vi "Scope Settings Dialog.vi"(11 "Scope Parameters":T1[](array[typedef]) {"Max input frequency" format="%#_6p Hz"; "Input impedance" items=["1 mega ohm"=0, "50 ohms"=2]; "Vertical coupling" items=["AC", "DC", "Ground"]; "Reference position" format="%#_6g %%"; "Min sample rate" format=" %#_6p S/s"}) -> (3 "Scope Parameters out":T1[](array[typedef]) {"Input impedance" items=["1 mega ohm"=0, "50 ohms"=2]; "Vertical coupling" items=["AC", "DC", "Ground"]; "Reference position" format="%#_6g %%"; "Min sample rate" format=" %#_6p S/s"})   [LabVIEW 2021, in "PMIC Common.lvlib"]
uses:
  PMIC Common.lvlib
  controls/UI Scope Parameters.ctl
panel:
  # "Horizontal"
  # "Vertical"
  # "Horizontal"
  # "Vertical"
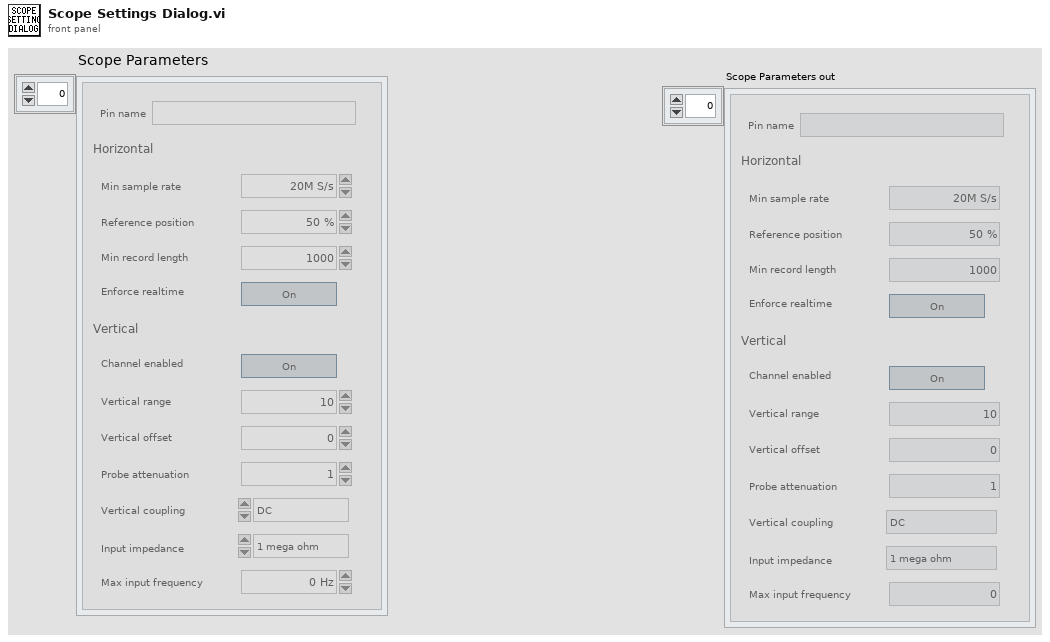
[diagram p1: front panel]
types:
  T1 = typedef "PMIC Common.lvlib/UI Scope Parameters.ctl" = cluster{"Pin name":string, "Vertical range":dbl, "Vertical offset":dbl, "Probe attenuation":dbl, "Vertical coupling":i32, "Channel enabled":bool, "Input impedance":u32, "Max input frequency":dbl, "Min sample rate":dbl, "Reference position":dbl, "Min record length":i32, "Enforce realtime":bool}
  T2 = enum32{"Invalid", "Standard", "Closed", "Hidden", "Minimized", "Maximized"}
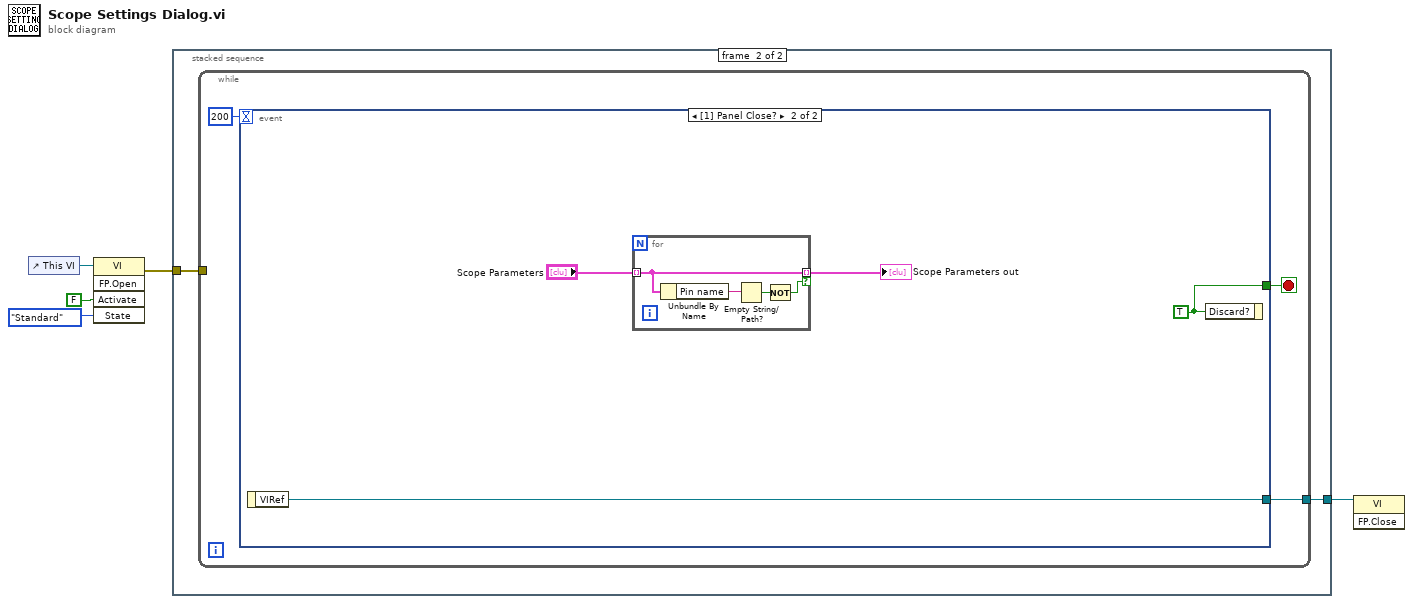
[diagram p0: block diagram]
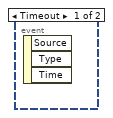
[diagram p3: hidden frame]
diagram:
  n1 = control-ref of="This VI"() -> (w5:refnum<vi>)
  n2 = invoke class="VI" method="FP.Open"(reference=w5, "Activate"=FALSE ("Activate?"), "State"=T2."Standard") -> (error out=w2:errorcluster)  [unwired: 2 in, 4 out]
  n3 = stacked-sequence {
    tunnel: w2 -> [_ w7]
    tunnel: [_ w6] -> w1
    frame #0 {
    }
    frame #1 {
      n4 = while {
        tunnel: [w8] -> w6
        tunnel: w7 -> [_]
        stop <- w10 stop-if-true
        n5 = event shown="[1] Panel Close?" {
          selector: _ -> [_ _]
          dyn-events: _ -> [_ _]
          timeout: 200 -> [_ _]
          tunnel: [_ w13] -> w10
          tunnel: [_ w14] -> w8
          event Timeout {
            n6 = event-data() -> ()  [unwired: 1 in, 3 out]
          }
          event Panel Close? {
            w13 = TRUE ("Discard?")
            n7 = event-data() -> ("VIRef"=w14:refnum<vi>)  [unwired: 1 in]
            n8 = for {
              tunnel: "Scope Parameters" -> [w16] mode=indexing
              tunnel: [w16] -> w11 mode=indexing if=w15
              n9 = Unbundle By Name(w16) -> ("Pin name"=w18:string)
              n10 = Empty String/Path?(string/path=w18) -> (empty?=w17:bool)
              n11 = Not(x=w17) -> (.not. x?=w15:bool)
            }
            "Scope Parameters out" <- w11
            n12 = event-data("Discard?"=w13) -> ()  [unwired: 1 in, 1 out]
          }
        }
      }
    }
  }
  n13 = invoke class="VI" method="FP.Close"(reference=w1) -> ()  [unwired: 2 in, 3 out]
